vi "Read configuration.vi"(8 "error in":errorcluster, 11 "Temperature Chamber Model editor node in":refnum<class "Temperature Chamber Model editor node.lvclass">) -> (0 "error out":errorcluster, 2 "configuration":refnum<class "NISE_CEF_serializable configuration.lvclass">, 3 "Temperature Chamber Model editor node out":refnum<class "Temperature Chamber Model editor node.lvclass">)   [LabVIEW 2013, in "Temperature Chamber Model editor node.lvclass"]
uses:
  Temperature Chamber Model editor node.lvclass
  <vilib>/NI/Configuration Framework/serializable configuration/NISE_CEF_serializable configuration.lvclass
  Temperature Chamber Model editor node.lvclass/Temperature Chamber Model editor node.ctl
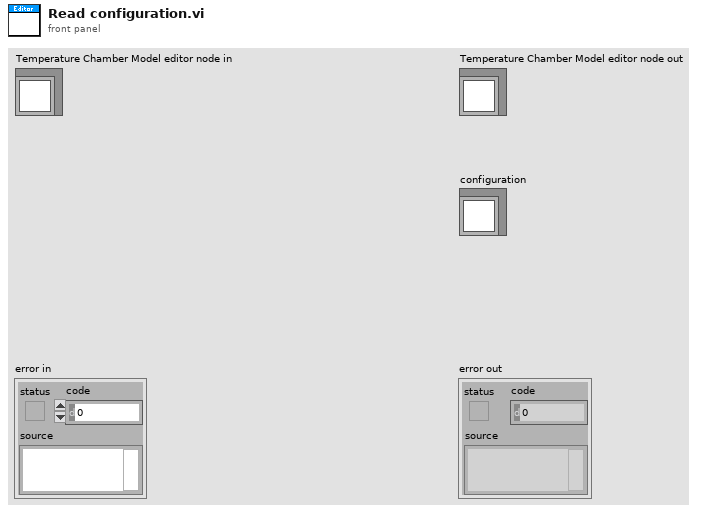
[diagram p1: front panel]
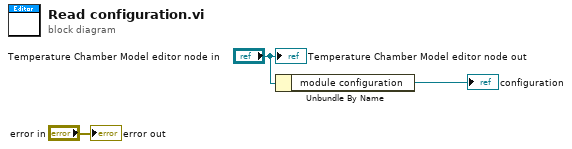
[diagram p0: block diagram]
diagram:
  n1 = Unbundle By Name("Temperature Chamber Model editor node in") -> ("module configuration"=→"configuration":refnum<class "Temperature Chamber Model configuration.lvclass">)
  "error out" <- "error in"
  "Temperature Chamber Model editor node out" <- "Temperature Chamber Model editor node in"
